vi "Determine Clicked Array Element Index - Test For Array Element Gap.vi"(0 "Array Reference":refnum<vi>, 5 "Array Property.Bounds.Width":u32, 7 "Un-gapped left coordinates":i32[](array[numeric]), 9 "Gapped left coordinates":i32[](array[numeric]), 11 "error in (no error)":errorcluster, 12 "Un-gapped top coordinates":i32[](array[numeric]), 13 "Gapped top coordinates":i32[](array[numeric])) -> (4 "dup Array Reference":refnum<vi>, 6 "Array has element gap?":bool, 8 "Column Left Coordinates":i32[](array[numeric]), 10 "Row Top Coordinates":i32[](array[numeric]), 15 "error out":errorcluster)   [LabVIEW 2015]
doc: "Determine Clicked Array Element Index - Test For Array Element Gap.vi\n\nDescription:\nThis VI determines if the array specified by the Array Reference input has an element gap displayed and outputs either the gapped or un-gapped coordinates accordingly.\n\nInputs:\nArray Reference - Reference to the array to operate on.\n\nArray Properties.Bounds.Width - The width of the array when the scrollbars, index display, label and caption are hidden.\n\nUn-gapped left coordinates - The left coordinates of each column with no element gap accounted for.\n\nGapped left coordinates - The left coordinates of each column with element gap accounted for.\n\nUn-gapped top coordinates - The top coordinates of each row with no element gap accounted for.\n\nGapped top coordinates - The top coordinates of each row with element gap accounted for.\n\nerror in - Standard error cluster.\n\nOutputs:\ndup Array Reference - Dup reference to the array to operate on.\n\nArray has element gap? - Indicates if the array has an element gap displayed or not.\n\nColumn left coordinates - The left coordinates of all columns displayed in the array.\n\nRow Top coordinates - The top coordinates of all rows displayed in the array.\n\nerror out - Standard error cluster.\n\nDeveloped By:\nMark.ridgley\nMark.Ridgley_LabVIEW.Developer@comcast.net"
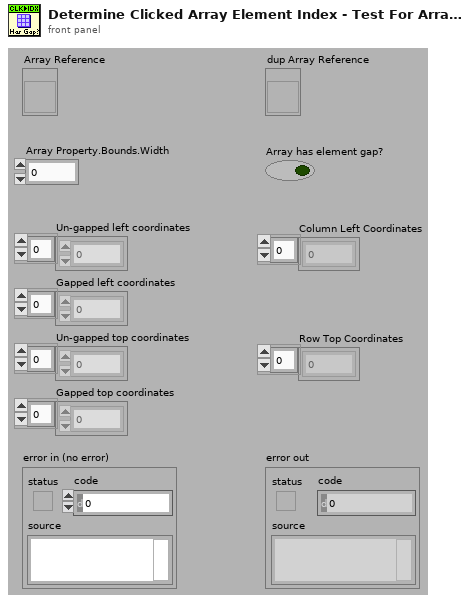
[diagram p1: front panel]
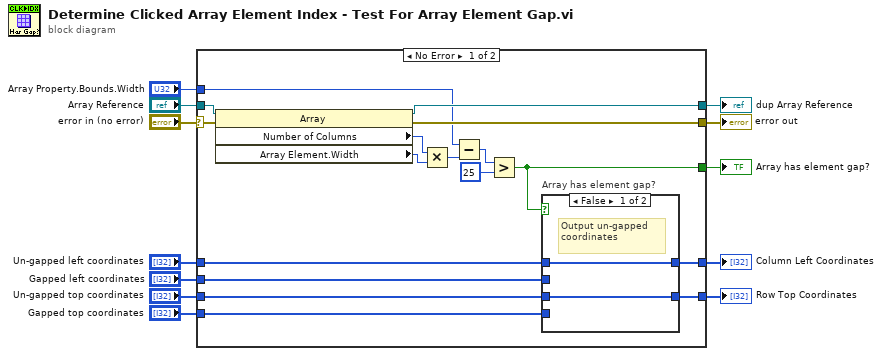
[diagram p0: block diagram]
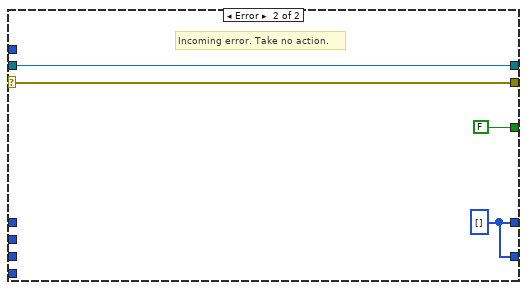
[diagram p3: hidden frame]
diagram:
  n1 = case shown="No Error" "error in (no error)" {
    selector: "error in (no error)" -> [w21 w36]
    tunnel: [w15 FALSE] -> w12
    tunnel: "Array Reference" -> [w26 w37]
    tunnel: [w23 w36] -> w10
    tunnel: [w22 w37] -> w9
    tunnel: "Array Property.Bounds.Width" -> [w20 _]
    tunnel: "Un-gapped left coordinates" -> [w19 _]
    tunnel: "Gapped left coordinates" -> [w18 _]
    tunnel: "Un-gapped top coordinates" -> [w17 _]
    tunnel: "Gapped top coordinates" -> [w16 _]
    tunnel: [w14 w34] -> w2
    tunnel: [w13 w34] -> w1
    frame No Error {
      n2 = property class="Array"(reference=w26, error in=w21) -> (reference out=w22:refnum<vi>, error out=w23:errorcluster, "Number of Columns"=w25:u32, "Array Element.Width"=w24:u32)
      n3 = Multiply(x=w25, y=w24) -> (x*y=w27:u32)
      n4 = Subtract(x=w20, y=w27) -> (x-y=w28:u32)
      n5 = Greater?(x=w28, y=u32 25) -> (0:w15:bool)
      n6 = case "Array has element gap?" shown="False" w15 {
        tunnel: w18 -> [_ w33]
        tunnel: [w31 w33] -> w14
        tunnel: w19 -> [w31 _]
        tunnel: w17 -> [w30 _]
        tunnel: [w30 w32] -> w13
        tunnel: w16 -> [_ w32]
        frame False {
          # "Output un-gapped\ncoordinates"
        }
        frame True {
          # "Output gapped\ncoordinates"
        }
      }
    }
    frame Error {
      w34 = i32[] [] ("Gapped left coordinates")
      # "Incoming error. Take no action."
    }
  }
  "Array has element gap?" <- w12
  "dup Array Reference" <- w9
  "error out" <- w10
  "Column Left Coordinates" <- w2
  "Row Top Coordinates" <- w1
